vi "Build Connection String.vi"(0 "Database Selector":T1, 1 "Server Address":string, 2 "Port":u32=3306, 5 "Driver":string, 7 "Username":string, 9 "Password":string, 11 "error in (no error)":errorcluster, 12 "ULD FIle or Connection String":bool, 13 "Schema Name":string, 14 "UDL Path":path) -> (4 "Connection String":string, 15 "error out (no error)":errorcluster)   [LabVIEW 2020]
uses:
  ctl/Database Selector.ctl
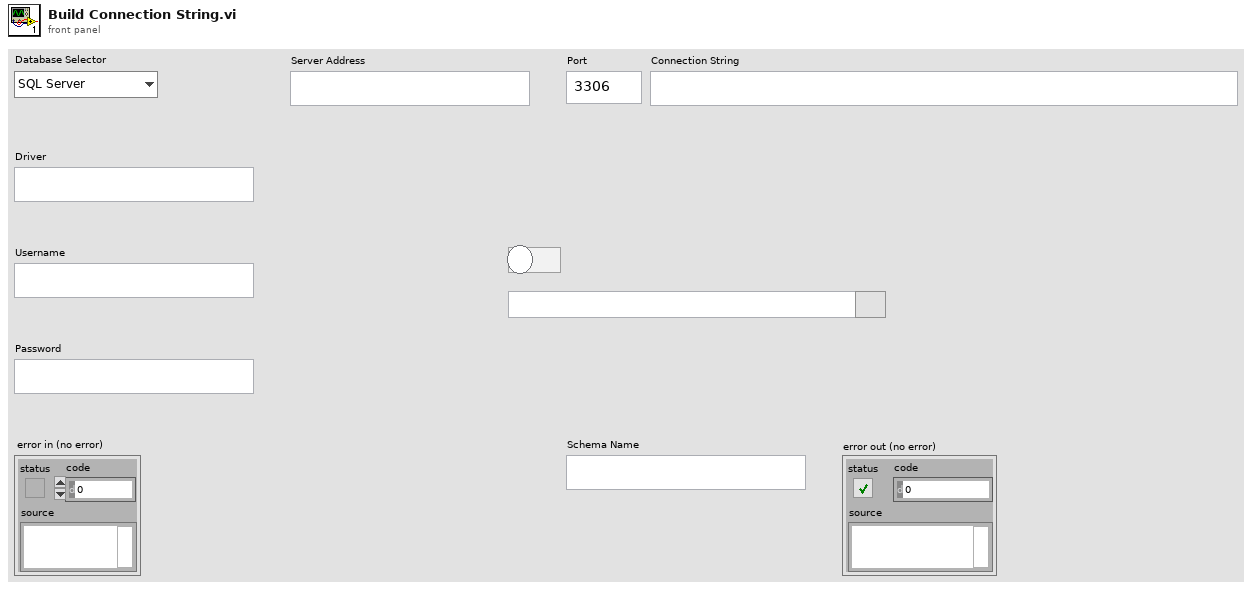
[diagram p1: front panel]
types:
  T1 = typedef "Database Selector.ctl" = enum16{"SQL Server", "MYSQL"}
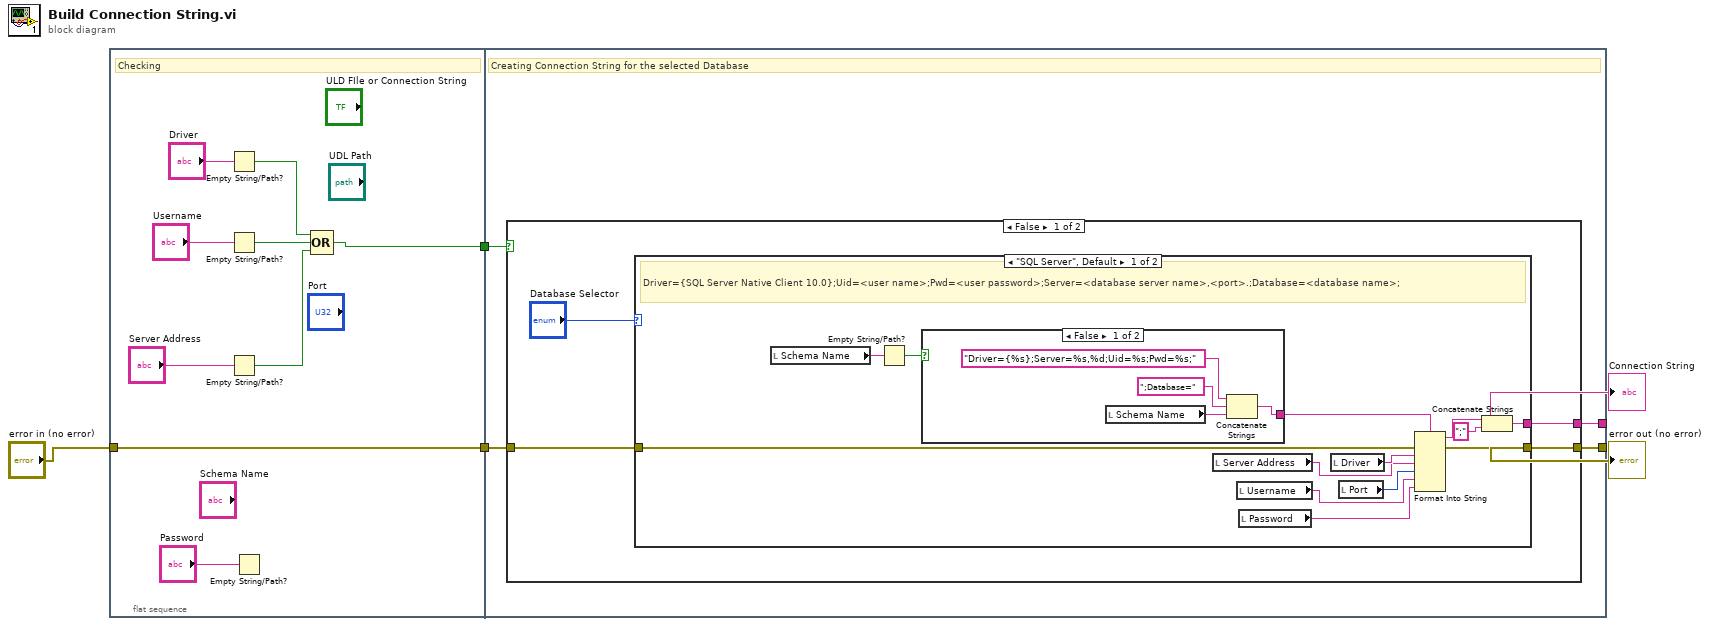
[diagram p0: block diagram]
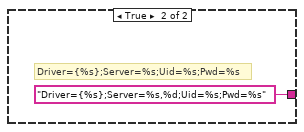
[diagram p2: hidden frame]
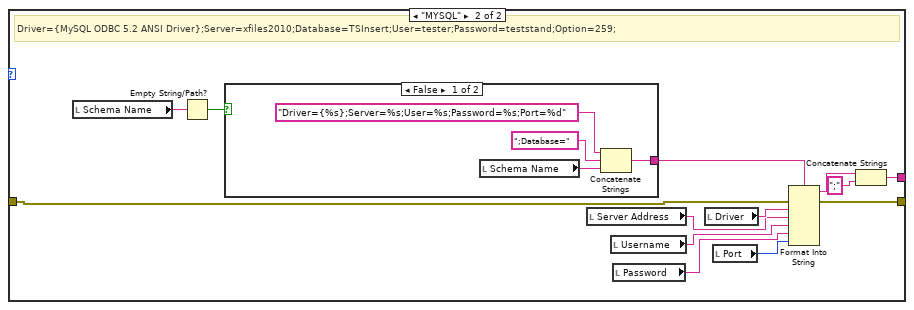
[diagram p3: hidden frame]
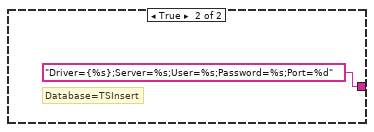
[diagram p4: hidden frame]
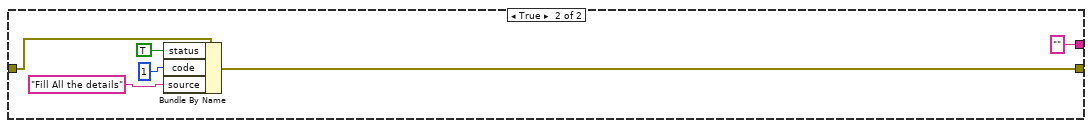
[diagram p5: hidden frame]
diagram:
  n1 = flat-sequence {
    tunnel: [w7] -> w5
    tunnel: [w6] -> w4
    tunnel: "error in (no error)" -> [w6]
    tunnel: w5 -> [w18]
    tunnel: w4 -> [w17]
    tunnel: [w16] -> w2
    tunnel: [w15] -> w1
    frame #0 {
      # "Checking"
      n2 = Empty String/Path?(string/path="Driver") -> (empty?=w10:bool)
      n3 = Empty String/Path?(string/path="Username") -> (empty?=w9:bool)
      n4 = Empty String/Path?(string/path="Server Address") -> (empty?=w8:bool)
      n5 = Empty String/Path?(string/path="Password") -> ()  [unwired: 1 out]
      n6 = Compound Arithmetic op=OR(w10, w9, w8) -> (w7:bool)
    }
    frame #1 {
      # "Creating Connection String for the selected Database"
      n7 = case shown="False" w18 {
        tunnel: w17 -> [w21 w64]
        tunnel: [w19 w60] -> w16
        tunnel: [w20 ""] -> w15
        frame False {
          n8 = case shown="\"SQL Server\", Default" "Database Selector" {
            tunnel: w21 -> [w28 w41]
            tunnel: [w26 w43] -> w20
            tunnel: [w27 w42] -> w19
            frame "SQL Server", Default {
              # "Driver={SQL Server Native Client 10.0};Uid=<user name>;Pwd=<user password>;Server=<database server name>,<port>.;Database=<database name>;"
              n9 = local read "Schema Name"() -> (w33:string)
              n10 = Empty String/Path?(string/path=w33) -> (empty?=w31:bool)
              n11 = case shown="False" w31 {
                tunnel: [w36 "Driver={%s};Server=%s,%d;Uid=%s;Pwd=%s" ("format string")] -> w32
                frame False {
                  n12 = local read "Schema Name"() -> (w37:string)
                  n13 = Concatenate Strings("Driver={%s};Server=%s,%d;Uid=%s;Pwd=%s;" ("format string"), ";Database=" ("string"), w37) -> (w36:string)
                }
                frame True {
                  # "Driver={%s};Server=%s;Uid=%s;Pwd=%s"
                }
              }
              n14 = local read "Server Address"() -> (w34:string)
              n15 = local read "Username"() -> (w24:string)
              n16 = local read "Password"() -> (w23:string)
              n17 = local read "Driver"() -> (w35:string)
              n18 = local read "Port"() -> (w25:u32)
              n19 = Format Into String(format string=w32, error in=w28, w35, w34, w25, w24, w23) -> (resulting string=w30:string, error out=w27:errorcluster)  [unwired: 1 in]
              n20 = Concatenate Strings(w30, ";" ("string")) -> (w26:string)
            }
            frame "MYSQL" {
              # "Driver={MySQL ODBC 5.2 ANSI Driver};Server=xfiles2010;Database=TSInsert;User=tester;Password=teststand;Option=259;"
              n21 = local read "Schema Name"() -> (w51:string)
              n22 = Empty String/Path?(string/path=w51) -> (empty?=w46:bool)
              n23 = case shown="False" w46 {
                tunnel: [w54 "Driver={%s};Server=%s;User=%s;Password=%s;Port=%d" ("format string")] -> w50
                frame False {
                  n24 = local read "Schema Name"() -> (w55:string)
                  n25 = Concatenate Strings("Driver={%s};Server=%s;User=%s;Password=%s;Port=%d" ("format string"), ";Database=" ("string"), w55) -> (w54:string)
                }
                frame True {
                  # "Database=TSInsert"
                }
              }
              n26 = local read "Server Address"() -> (w52:string)
              n27 = local read "Username"() -> (w49:string)
              n28 = local read "Password"() -> (w48:string)
              n29 = local read "Driver"() -> (w53:string)
              n30 = local read "Port"() -> (w47:u32)
              n31 = Format Into String(format string=w50, error in=w41, w53, w52, w49, w48, w47) -> (resulting string=w45:string, error out=w42:errorcluster)  [unwired: 1 in]
              n32 = Concatenate Strings(w45, ";" ("string")) -> (w43:string)
            }
          }
        }
        frame True {
          n33 = Bundle By Name(cluster=w64, "status"=TRUE, "code"=1, "source"="Fill All the details") -> (w60:errorcluster)
        }
      }
    }
  }
  "error out (no error)" <- w2
  "Connection String" <- w1
